vi "J1939 Data Lookup Table Initialize.vi"(8 "error in (no error)":errorcluster, 10 "initial values":dbl[](array[numeric]), 11 "channel information":T1) -> (0 "error out":errorcluster {"code" min=0 max=0}, 3 "vi reference":T3)   [LabVIEW 2013, in "J1939.lvlib"]
uses:
  J1939.lvlib
  J1939 Data Lookup Table Reference.ctl
  API Types/Scaling Initialization.ctl
  Users/Benjamin/Desktop/Tag bus J1939/J1939/RT Driver/SubVIs/CD Conversion Lookup Table Parameters Cluster.ctl
  J1939 Data Lookup Table Action.ctl
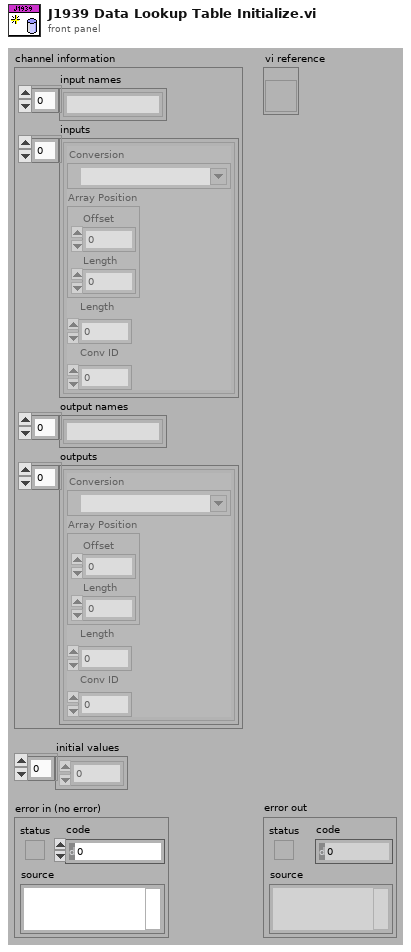
[diagram p1: front panel]
types:
  T1 = typedef "J1939.lvlib/scaling initialization.ctl" = cluster{"input names":string[], "inputs":T2[], "output names":string[], "outputs":T2[]}
  T2 = typedef "J1939.lvlib/CD Conversion Lookup Table Parameters Cluster.ctl" = cluster{"Conversion":refnum<k21>, "Array Position":cluster{"Offset":u32, "Length":u32}, "Length":u32, "Conv ID":u32}
  T3 = typedef "J1939.lvlib/J1939 Data Lookup Table Reference.ctl" = refnum<vi>
  T4 = typedef "J1939.lvlib/J1939 Data Lookup Table Action.ctl" = enum16{"Get All", "Set All", "Set Frame", "Get Frame", "Set Range", "Get Range"}
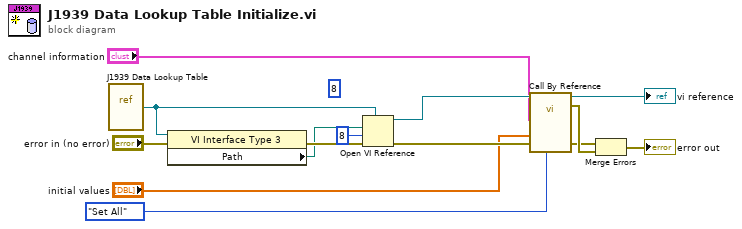
[diagram p0: block diagram]
diagram:
  (unwired) 8 ("options")
  n1 = vi-ref "J1939 Data Lookup Table.vi"() -> (w14:refnum<vi>)
  n2 = property class="VI Interface Type 3"(reference=w14, error in="error in (no error)") -> (error out=w12:errorcluster, "Path"=w4:path)  [unwired: 1 out]
  n3 = Open VI Reference(type specifier VI Refnum (for type only)=w14, vi path=w4, options=8, error in (no error)=w12) -> (vi reference=w11:refnum<vi>, error out=w7:errorcluster)  [unwired: 2 in]
  n4 = call-by-ref "?"(reference=w11, "command"=J1939_Data_Lookup_Table_Action."Set All", "error in (no error)"=w7, "Signals"="initial values", "scaling information"="channel information") -> (reference out=→"vi reference":refnum<vi>, error out=w10:errorcluster, 0:"error out"=w6:errorcluster)  [unwired: 7 in, 1 out]
  n5 = Merge Errors(w6, w10) -> (→"error out":errorcluster)
